vi "write_lockFile.vi"(6 "append?":bool, 7 "delimater":string=",", 9 "1-D Array String":string[](array[string])=["5", "5", "5", "5"], 11 "file path (use dialog)":path) -> ()   [LabVIEW 2022 SP3]
panel:
  in  "error in":errorcluster
  out "error out":errorcluster
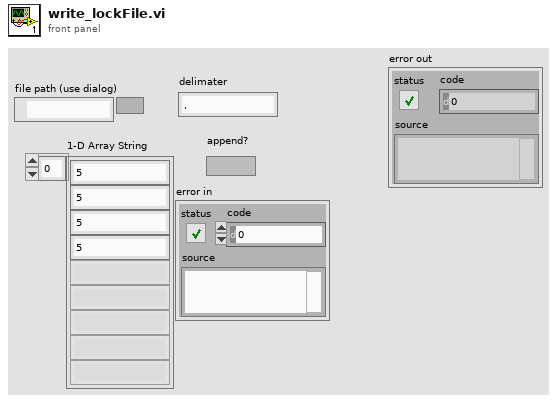
[diagram p1: front panel]
types:
  T1 = enum16{"open", "replace", "create", "open or create", "replace or create", "replace or create with confirmation"}
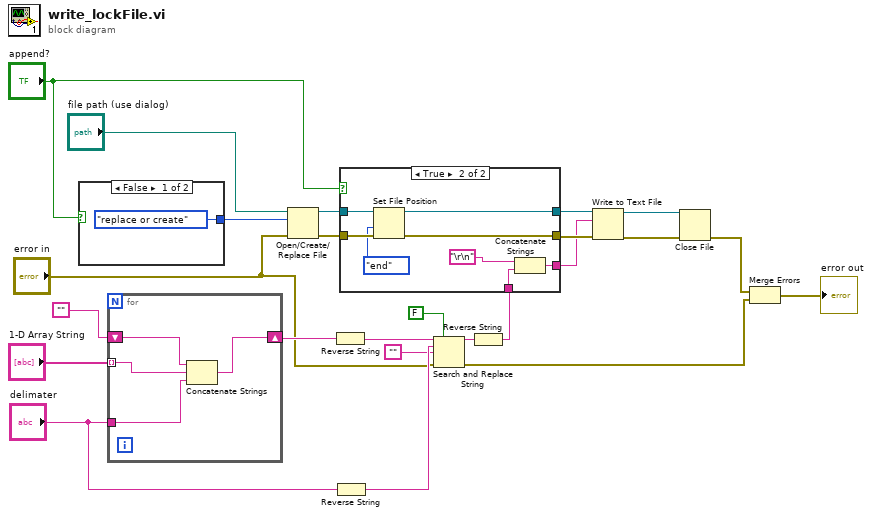
[diagram p0: block diagram]
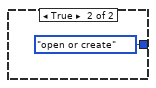
[diagram p3: hidden frame]
diagram:
  n1 = case shown="False" "append?" {
    tunnel: [T1."replace or create" ("operation (0:open)") T1."open or create" ("operation (0:open)")] -> w24
    frame False {
    }
    frame True {
    }
  }
  n2 = for {
    tunnel: "1-D Array String" -> [w29] mode=indexing
    shift-right: [w27] -> w15
    shift-left: "" -> [w30]
    tunnel: "delimater" -> [w28]
    n3 = Concatenate Strings(w30, w29, w28) -> (w27:string)
  }
  n4 = Open/Create/Replace File(file path (use dialog)="file path (use dialog)", error in="error in", operation (0:open)=w24) -> (refnum out=w19:refnum<file>, error out=w20:errorcluster)  [unwired: 3 in, 1 out]
  n5 = Reverse String(1:w15) -> (0:w13:string)
  n6 = Reverse String(1:"delimater") -> (0:w11:string)
  n7 = Search and Replace String(replace all?=FALSE ("replace all? (F)"), input string=w13, search string=w11, replace string="", error in="error in") -> (result string=w3:string, error out=w6:errorcluster)  [unwired: 3 in, 2 out]
  n8 = Reverse String(1:w3) -> (0:w2:string)
  n9 = case shown="True" "append?" {
    tunnel: w20 -> [w32 w41]
    tunnel: w19 -> [w33 w40]
    tunnel: [w32 w38] -> w17
    tunnel: [w33 w37] -> w16
    tunnel: w2 -> [w31 w35]
    tunnel: [w31 w34] -> w1
    frame False {
    }
    frame True {
      n10 = Set File Position(refnum=w40, from (0:start)=enum16{"start", "end", "current"}."end", error in=w41) -> (refnum out=w37:refnum<file>, error out=w38:errorcluster)  [unwired: 1 in]
      n11 = Concatenate Strings("\r\n", w35) -> (w34:string)
    }
  }
  n12 = Write to Text File(file (use dialog)=w16, text=w1, error in=w17) -> (refnum out=w8:refnum<file>, error out=w9:errorcluster)  [unwired: 1 in, 1 out]
  n13 = Close File(refnum=w8, error in=w9) -> (error out=w5:errorcluster)  [unwired: 1 out]
  n14 = Merge Errors(w5, w6) -> (→"error out":errorcluster)
